vi "Read Data.vi"(8 "error in (no error)":errorcluster, 10 "Count":i32, 11 "TCP Stream in":refnum<class "TCP Stream.lvclass">) -> (0 "error out":errorcluster, 2 "Data":string, 3 "TCP Stream out":refnum<class "TCP Stream.lvclass">)   [LabVIEW 2020, in "Stream-TCP.lvlib" / "TCP Stream.lvclass"]
uses:
  TCP Stream.lvclass
  TCP Stream.lvclass/TCP Stream.ctl
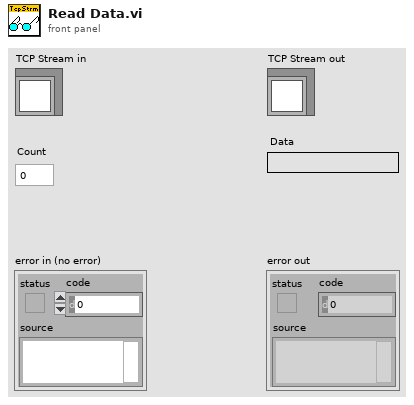
[diagram p1: front panel]
types:
  T1 = enum16{"Standard", "Buffered", "CRLF", "Immediate"}
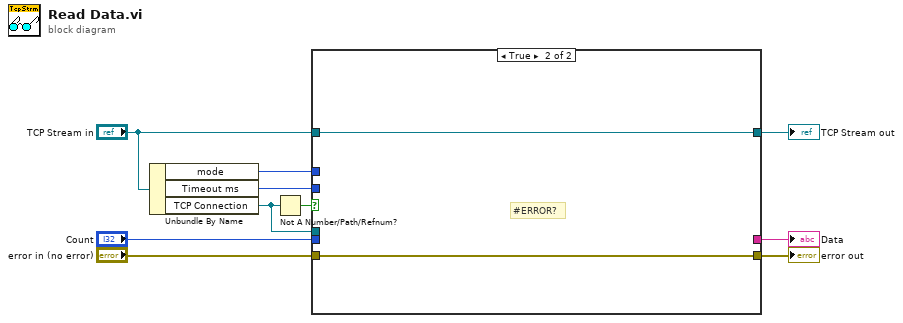
[diagram p0: block diagram]
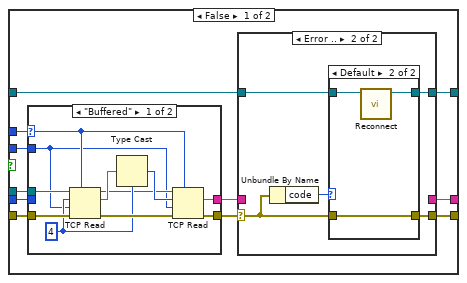
[diagram p2: hidden frame]
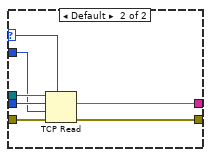
[diagram p5: hidden frame]
diagram:
  n1 = Unbundle By Name("TCP Stream in") -> ("mode"=w7:T1, "Timeout ms"=w6:i32, "TCP Connection"=w2:refnum<k5>)
  n2 = Not A Number/Path/Refnum?(number/path/refnum=w2) -> (NaN/Path/Refnum?=w1:bool)
  n3 = case shown="True" w1 {
    tunnel: "Count" -> [w21 _]
    tunnel: "TCP Stream in" -> [w19 w54]
    tunnel: [w18 w54] -> w8
    tunnel: w7 -> [w17 _]
    tunnel: w6 -> [w16 _]
    tunnel: [w14 _] -> w5
    tunnel: "error in (no error)" -> [w13 w53]
    tunnel: [w12 w53] -> w3
    tunnel: w2 -> [w11 _]
    frame False {
      n4 = case shown="\"Buffered\"" w17 {
        selector: w17 -> [w38 w46]
        tunnel: w11 -> [w44 w52]
        tunnel: w13 -> [w43 w51]
        tunnel: w21 -> [_ w50]
        tunnel: [w36 w49] -> w20
        tunnel: [w37 w48] -> w15
        tunnel: w16 -> [w35 w47]
        frame "Buffered" {
          w41 = 4
          n5 = TCP Read(connection ID=w44, bytes to read=w41, error in (no error)=w43, 7:w38, 9:w35) -> (connection ID out=w39:refnum<k5>, data out=w42:string, error out=w45:errorcluster)
          n6 = Type Cast(type=w41, x=w42) -> (*(type *) &x=w40:i32)
          n7 = TCP Read(connection ID=w39, bytes to read=w40, error in (no error)=w45, 7:w38, 9:w35) -> (data out=w37:string, error out=w36:errorcluster)  [unwired: 1 out]
        }
        frame Default {
          n8 = TCP Read(connection ID=w52, bytes to read=w50, error in (no error)=w51, 7:w46, 9:w47) -> (data out=w48:string, error out=w49:errorcluster)  [unwired: 1 out]
        }
      }
      n9 = case shown="Error .." w20 {
        selector: w20 -> [w22 w29]
        tunnel: [w22 w28] -> w12
        tunnel: w19 -> [w24 w27]
        tunnel: [w24 w26] -> w18
        tunnel: w15 -> [w23 _]
        tunnel: [w23 _] -> w14
        frame No Error {
        }
        frame Error {
          n10 = Unbundle By Name(w29) -> ("code"=w25:i32)
          n11 = case shown="Default" w25 {
            tunnel: w27 -> [w31 w34]
            tunnel: [w31 w33] -> w26
            tunnel: w29 -> [w30 w32]
            tunnel: [w30 w32] -> w28
            frame 56 {
            }
            frame Default {
              n12 = call "Reconnect.vi"("TCP Stream in"=w34) -> ("TCP Stream out"=w33:refnum<class "TCP Stream.lvclass">)  [unwired: 9 in, 1 out]
            }
          }
        }
      }
    }
    frame True {
      # "#ERROR?"
    }
  }
  "error out" <- w3
  "TCP Stream out" <- w8
  "Data" <- w5
